vi "Receive_Packet.vi"(5 "Packet? (t)":bool=TRUE, 6 "clear_timeout_error (f)":bool, 7 "mode (standard)":T1(ring), 8 "error in (no error)":errorcluster, 10 "Offset/Bufsize":u32, 11 "Socket.TCP in":refnum<class "Socket.TCP.lvclass">) -> (0 "error out":errorcluster, 1 "bytes_read":i32, 2 "data_out":string, 3 "Socket.TCP out":refnum<class "Socket.TCP.lvclass">)   [LabVIEW 2014, in "Socket.lvlib" / "Socket.TCP.lvclass"]
doc: "socket.tcp.Receive (mode, bufsize, [clear_timeout_error]) Waits for the timeout period in ms and returns bytes received or timeout error.\n\nenum mode\n Standard: Waits until all bytes in bufsize arrive or until timeout. If timeout occurs, returns the bytes read so far and reports timeout error.\n Buffered: Waits until all bytes in bufsize arrive or until timeout. If timeout occurs, returns no bytes and reports timeout error\n CRLF: Waits until all bytes in bufsize arrive or until a carriage return (CR) followed by a linefeed (LF) or until timeout. Returns all bytes including the CR and LF. If timeout occurs before CRLF, returns no bytes and a timeout error.\n Immediate: Waits until any bytes in bufsize arrive. Only reports a timeout errror if no bytes arrive.\n\nu32 bufsize is the amount of bytes the receiver will wait for as determined by mode. If bufsize = 0, the incoming bytes are assumed to be a TCP packet and the first two bytes will be used to determine the size of the following packet to be received.\n\nbool clear_timeout_error optional input to clear the timeout error before exiting the method. This is used when looping receive to check for loop exit conditions."
uses:
  Socket.TCP.lvclass
  Socket.TCP.lvclass/Socket.TCP.ctl
  Socket.Base/Socket.Base.lvclass/Socket.Base.ctl
  Accessors/Read tcp _refnum.vi
  Socket.Base/Accessors/Read timeout.vi
panel:
  # "If Packet? is TRUE, Offset is the number of bytes from the data start where the 2-byte data length will be found."
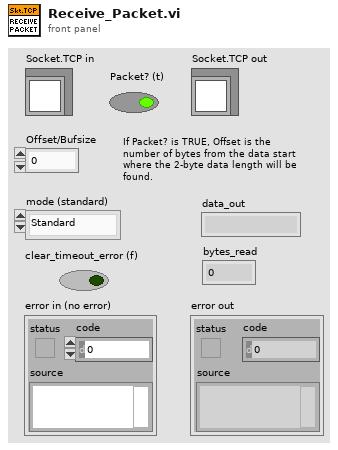
[diagram p1: front panel]
types:
  T1 = enum16{"Standard", "Buffered", "CRLF", "Immediate"}
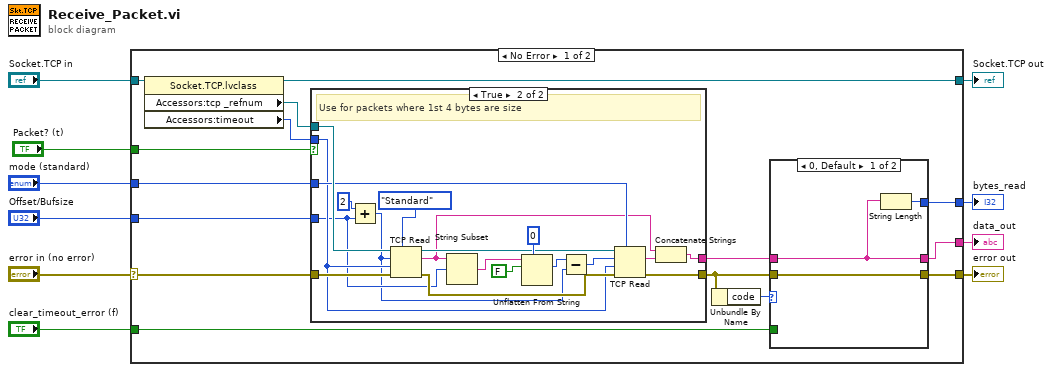
[diagram p0: block diagram]
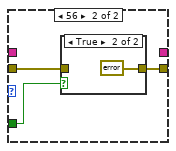
[diagram p2: hidden frame]
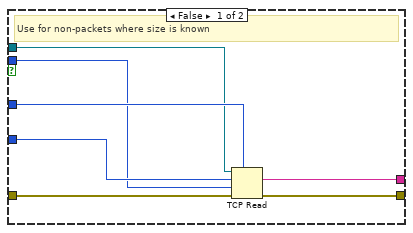
[diagram p4: hidden frame]
diagram:
  n1 = case shown="No Error" "error in (no error)" {
    selector: "error in (no error)" -> [w19 w61]
    tunnel: [w18 w61] -> w9
    tunnel: [w24 w60] -> w7
    tunnel: "Socket.TCP in" -> [w25 w60]
    tunnel: "mode (standard)" -> [w23 _]
    tunnel: "Offset/Bufsize" -> [w22 _]
    tunnel: "clear_timeout_error (f)" -> [w17 _]
    tunnel: [w14 _] -> w3
    tunnel: [w13 _] -> w2
    tunnel: "Packet? (t)" -> [w12 _]
    frame No Error {
      n2 = property class="Socket.TCP.lvclass"(reference=w25) -> (reference out=w24:refnum<class "Socket.TCP.lvclass">, "Accessors:tcp _refnum"=w20:refnum<k5>, "Accessors:timeout"=w21:i32)  [unwired: 1 in, 1 out]
      n3 = case shown="True" w12 {
        tunnel: w23 -> [w37 w56]
        tunnel: w21 -> [w34 w48]
        tunnel: w20 -> [w36 w57]
        tunnel: w19 -> [w40 w55]
        tunnel: [w39 w54] -> w16
        tunnel: [w38 w42] -> w11
        tunnel: w22 -> [w35 w46]
        frame False {
          # "Use for non-packets where size is known"
          n4 = TCP Read(connection ID=w36, bytes to read=w35, error in (no error)=w40, 7:w37, 9:w34) -> (data out=w38:string, error out=w39:errorcluster)  [unwired: 1 out]
        }
        frame True {
          # "Use for packets where 1st 4 bytes are size"
          n5 = Add(x=u32 2, y=w46) -> (x+y=w45:u32)
          n6 = TCP Read(connection ID=w57, bytes to read=w45, error in (no error)=w55, 7:T1."Standard" ("mode (standard)"), 9:w48) -> (connection ID out=w43:refnum<k5>, data out=w41:string, error out=w59:errorcluster)
          n7 = String Subset(string=w41, offset (0)=w46) -> (substring=w50:string)  [unwired: 1 in]
          n8 = Unflatten From String(type=u16 0 ("default (0 I32)"), binary string=w50, data includes array or string size? (T)=FALSE) -> (value=w47:u16)  [unwired: 2 in, 2 out]
          n9 = Subtract(x=w47, y=w45) -> (x-y=w44:u32)
          n10 = TCP Read(connection ID=w43, bytes to read=w44, error in (no error)=w59, 7:w56, 9:w48) -> (data out=w53:string, error out=w54:errorcluster)  [unwired: 1 out]
          n11 = Concatenate Strings(w41, w53) -> (w42:string)
        }
      }
      n12 = Unbundle By Name(w16) -> ("code"=w15:i32)
      n13 = case shown="0, Default" w15 {
        tunnel: w16 -> [w28 w31]
        tunnel: [w28 w30] -> w18
        tunnel: w11 -> [w26 _]
        tunnel: [w26 _] -> w13
        tunnel: [w27 _] -> w14
        tunnel: w17 -> [_ w29]
        frame 0, Default {
          n14 = String Length(string=w26) -> (length=w27:i32)
        }
        frame 56 {
          n15 = case shown="True" w29 {
            tunnel: w31 -> [w32 _]
            tunnel: [w32 errorcluster {"status"=FALSE, "code"=0, "source"=""} ("error constant")] -> w30
            frame False {
            }
            frame True {
            }
          }
        }
      }
    }
    frame Error {
    }
  }
  "error out" <- w9
  "Socket.TCP out" <- w7
  "bytes_read" <- w3
  "data_out" <- w2
